vi "Modbus Round Number.vi"(11 "Number":dbl) -> (3 "Rounded Number":dbl)   [LabVIEW 2020, in "Modbus.lvlib"]
uses:
  Modbus.lvlib
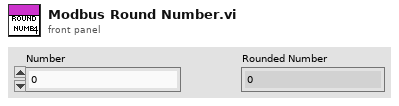
[diagram p1: front panel]
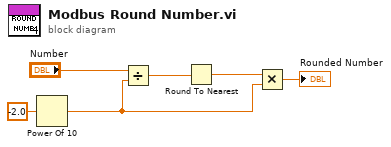
[diagram p0: block diagram]
diagram:
  n1 = Power Of 10(x=-2.0) -> (10^x=w4:dbl)
  n2 = Divide(x="Number", y=w4) -> (x/y=w3:dbl)
  n3 = Round To Nearest(number=w3) -> (nearest integer value=w5:dbl)
  n4 = Multiply(x=w5, y=w4) -> (x*y=→"Rounded Number":dbl)
